vi "CapacitiveTouch TouchInputEvents Example.vi"() -> ()   [LabVIEW 2012, in "Phidget Capacitive Touch.lvlib"]
uses:
  <instrlib>/Phidgets/Phidget Capacitive Touch/Phidget Capacitive Touch.lvlib
  <instrlib>/Phidgets/Phidget Capacitive Touch/Public/CapacitiveTouchStart.vi
  <instrlib>/Phidgets/Phidget Capacitive Touch/Public/CapacitiveTouchClose.vi
  <instrlib>/Phidgets/Phidget Common/Phidget Common.lvlib
panel:
  in  "stop 2":bool caption="stop"
  out "Is Touched":bool
  out "Touch Input Value":dbl caption="TouchInputValue"
  in  "stop":bool
  out "Serial Number Return":i32
  in  "Device Info":T1={"Serial Number"=-1, "Channel"=0, "Port"=0}
  out "error out":errorcluster
  # "Be sure to use this stop button to stop the program.\nIf you use the \"Abort Execution\" button, you will\nneed to use PhidgetResetLibrary.vi or restart Labview \nin order for any Phidgets to work."
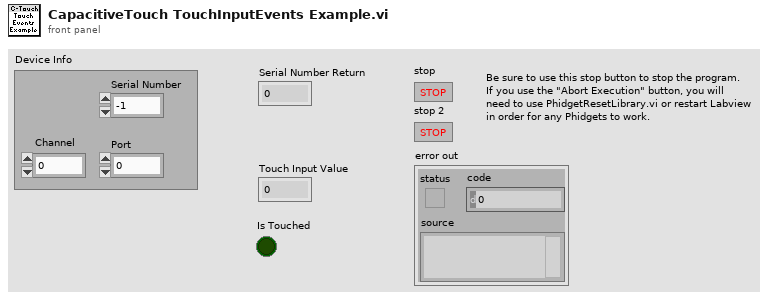
[diagram p1: front panel]
types:
  T1 = cluster{"Serial Number":i32, "Channel":i32, "Port":i32}
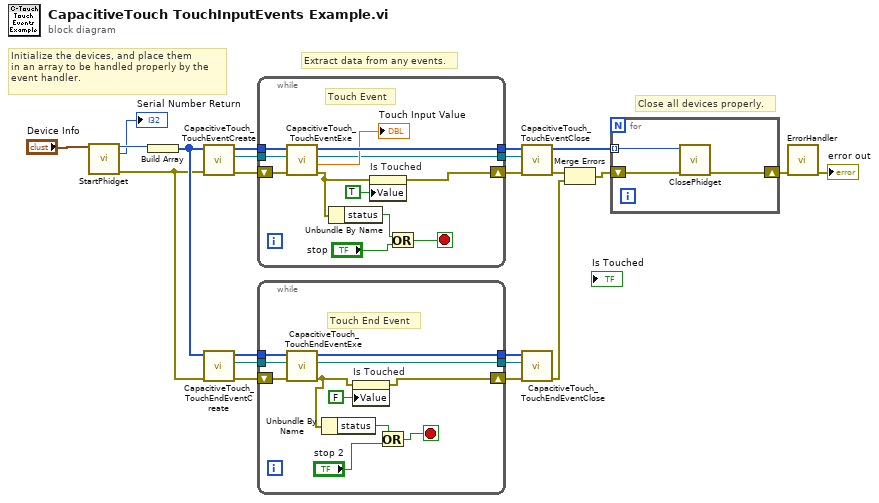
[diagram p0: block diagram]
diagram:
  # "Close all devices properly."
  # "Extract data from any events."
  # "Initialize the devices, and place them\nin an array to be handled properly by the\nevent handler."
  n1 = call-poly <instrlib>:"StartPhidget.vi"("Device Info"="Device Info") -> ("Phidget ID"=w15:u64, "Serial Number Return"=→"Serial Number Return":i32, "error out"=w4:errorcluster)  [unwired: 11 in, 1 out]
  n2 = Build Array(w15) -> (w5:u64[])
  n3 = call <instrlib>:"CapacitiveTouch_TouchEventCreate.vi"("error in (no error)"=w4, "Devices In"=w5) -> ("error out"=w17:errorcluster, "Event Registration Refnum"=w22:refnum<event-registration>, "Devices Out"=w23:u64[])  [unwired: 7 in]
  n4 = call <instrlib>:"CapacitiveTouch_TouchEndEventCreate.vi"("error in (no error)"=w4, "Devices In"=w5) -> ("error out"=w7:errorcluster, "Event Registration Refnum"=w10:refnum<event-registration>, "Devices Out"=w11:u64[])  [unwired: 7 in]
  n5 = while {
    tunnel: w23 -> [w35]
    tunnel: w22 -> [w32]
    tunnel: [w28] -> w19
    shift-right: [w26] -> w18
    shift-left: w17 -> [w34]
    tunnel: [w33] -> w13
    stop <- w27 stop-if-true
    # "Touch Event"
    n6 = call <instrlib>:"CapacitiveTouch_TouchEventExe.vi"("error in (no error)"=w34, "Event Registration Refnum In"=w32, "Devices In"=w35) -> ("error out"=w25:errorcluster, "Touch Value"=→"Touch Input Value":dbl, "Event Registration Refnum Out"=w28:refnum<event-registration>, "Devices Out"=w33:u64[])  [unwired: 2 in, 3 out]
    n7 = Unbundle By Name(w25) -> ("status"=w30:bool)
    n8 = property on="Is Touched" class="Bool (strict)"(error in=w25, "Value"=TRUE ("Is Touched")) -> (error out=w26:errorcluster)  [unwired: 1 in, 1 out]
    n9 = Or(x=w30, y="stop") -> (x .or. y?=w27:bool)
  }
  n10 = while {
    tunnel: w11 -> [w46]
    tunnel: w10 -> [w43]
    tunnel: [w42] -> w9
    shift-right: [w41] -> w8
    shift-left: w7 -> [w45]
    tunnel: [w44] -> w6
    stop <- w37 stop-if-true
    # "Touch End Event"
    n11 = call <instrlib>:"CapacitiveTouch_TouchEndEventExe.vi"("error in (no error)"=w45, "Event Registration Refnum In"=w43, "Devices In"=w46) -> ("error out"=w39:errorcluster, "Event Registration Refnum Out"=w42:refnum<event-registration>, "Devices Out"=w44:u64[])  [unwired: 3 in, 3 out]
    n12 = Unbundle By Name(w39) -> ("status"=w38:bool)
    n13 = property on="Is Touched" class="Bool (strict)"(error in=w39, "Value"=FALSE ("Is Touched")) -> (error out=w41:errorcluster)  [unwired: 1 in, 1 out]
    n14 = Or(x=w38, y="stop 2") -> (x .or. y?=w37:bool)
  }
  n15 = call <instrlib>:"CapacitiveTouch_TouchEventClose.vi"("error in (no error)"=w18, "Event Registration Refnum In"=w19, "Devices In"=w13) -> ("error out"=w3:errorcluster, "Devices Out"=w14:u64[])  [unwired: 7 in]
  n16 = call <instrlib>:"CapacitiveTouch_TouchEndEventClose.vi"("error in (no error)"=w8, "Event Registration Refnum In"=w9, "Devices In"=w6) -> ("error out"=w1:errorcluster)  [unwired: 7 in, 1 out]
  n17 = Merge Errors(w3, w1) -> (w2:errorcluster)
  n18 = for {
    tunnel: w14 -> [w47] mode=indexing
    shift-right: [w49] -> w21
    shift-left: w2 -> [w48]
    n19 = call-poly <instrlib>:"ClosePhidget.vi"("error in"=w48, "Device In"=w47) -> ("error out"=w49:errorcluster)  [unwired: 9 in]
  }
  n20 = call <instrlib>:"ErrorHandler.vi"("error in"=w21) -> ("error out"=→"error out":errorcluster)  [unwired: 9 in, 1 out]
